vi "Write Purge.vi"(8 "error in (no error)":errorcluster, 10 "Purge":T1, 11 "Potting Procedure in":refnum<class "Potting Procedure.lvclass">) -> (0 "error out":errorcluster, 3 "Potting Procedure out":refnum<class "Potting Procedure.lvclass">)   [LabVIEW 2017, in "Potting Procedure.lvclass"]
uses:
  Potting Procedure.lvclass
  Type Definitions/Purge.ctl
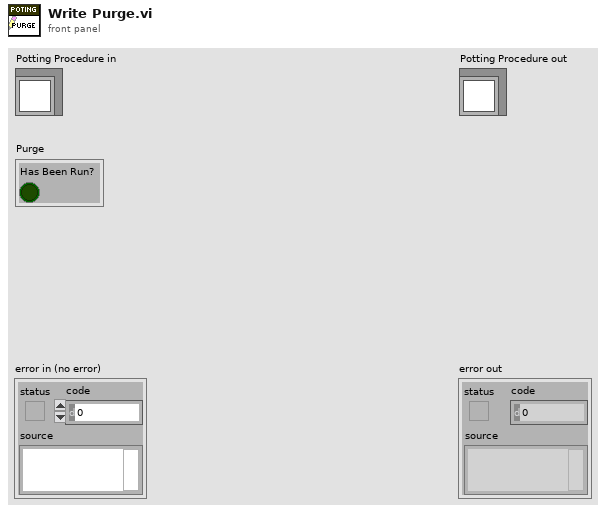
[diagram p1: front panel]
types:
  T1 = typedef "Purge.ctl" = cluster{"Has Been Run?":bool}
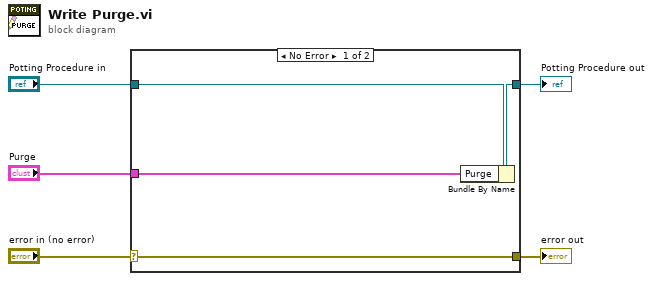
[diagram p0: block diagram]
diagram:
  n1 = case shown="No Error" "error in (no error)" {
    selector: "error in (no error)" -> [w9 w10]
    tunnel: [w9 w10] -> w4
    tunnel: [w7 w11] -> w2
    tunnel: "Potting Procedure in" -> [w8 w11]
    tunnel: "Purge" -> [w6 _]
    frame No Error {
      n2 = Bundle By Name(cluster=w8, "Purge"=w6) -> (w7:refnum<class "Potting Procedure.lvclass">)
    }
    frame Error {
    }
  }
  "error out" <- w4
  "Potting Procedure out" <- w2
